vi "Get Users.vi"(3 "error in (no error)":errorcluster, 5 "Database.lvlib:Data Store.lvclass":refnum<class "Data Store.lvclass">) -> (0 "error out":errorcluster, 1 "Array":T1[](array[typedef]), 2 "Database.lvlib:Data Store.lvclass 2":refnum<class "Data Store.lvclass">)   [LabVIEW 2011, in "Database.lvlib" / "Data Store.lvclass"]
uses:
  Data Store.lvclass
  User.ctl
  Data Store.lvclass/Data Store.ctl
  <vilib>/addons/database/_DB Variant To Data/Database Variant To Data.xnode
  <vilib>/addons/database/NI_Database_API.lvlib
  Database.lvlib
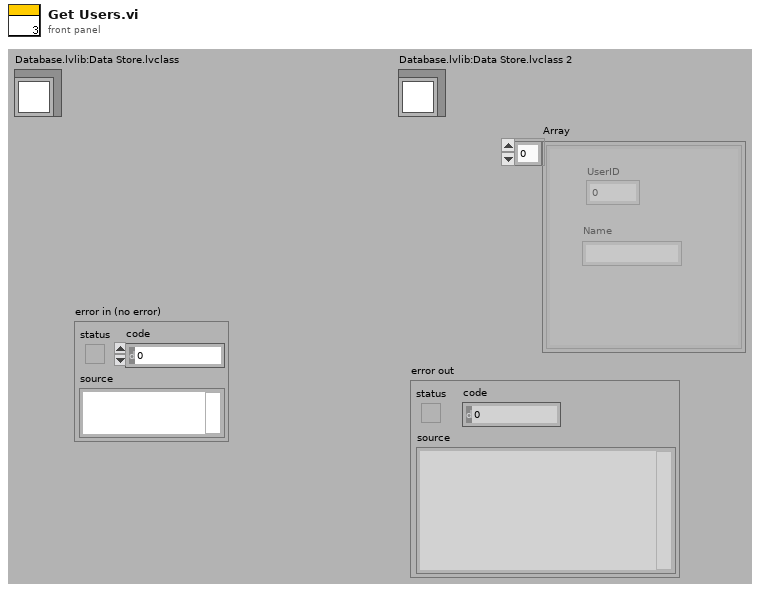
[diagram p1: front panel]
types:
  T1 = typedef "Database.lvlib/User.ctl" = cluster{"UserID":i32, "Name":string}
  T2 = typedef "NI_Database_API.lvlib/Conn ObjectReference.ctl" = refnum<k1>
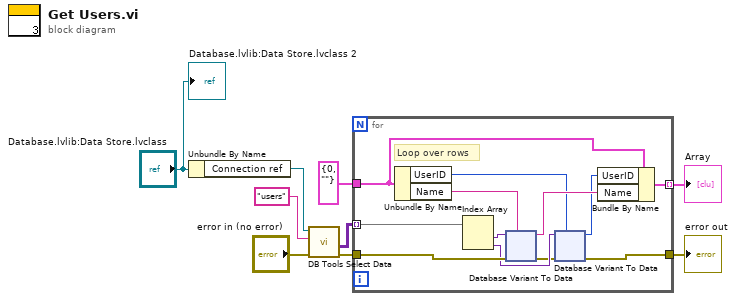
[diagram p0: block diagram]
diagram:
  n1 = Unbundle By Name("Database.lvlib:Data Store.lvclass") -> ("Connection ref"=w9:T2)
  n2 = call <vilib>:"DB Tools Select Data.vi"("error in (no error)"="error in (no error)", "table"="users", "connection reference"=w9) -> ("error out"=w6:errorcluster, "data"=w5:variant[][])  [unwired: 3 in, 1 out]
  n3 = for {
    tunnel: w6 -> [w19]
    tunnel: w5 -> [w21] mode=indexing
    tunnel: T1 {"UserID"=0, "Name"=""} ("Cluster") -> [w16]
    tunnel: [w14] -> w3 mode=indexing
    tunnel: [w15] -> w2
    # "Loop over rows"
    n4 = Unbundle By Name(w16) -> ("UserID"=w11:i32, "Name"=w13:string)
    n5 = Index Array(array=w21) -> (element #1=w20:variant, element #2=w18:variant)  [unwired: 2 in]
    n6 = xnode "Database Variant To Data"("database variant"=w20, "error in"=w19, "type"=w13) -> ("data"=w12:string, "error out"=w17:errorcluster)
    n7 = xnode "Database Variant To Data"("database variant"=w18, "error in"=w17, "type"=w11) -> ("data"=w10:i32, "error out"=w15:errorcluster)
    n8 = Bundle By Name(cluster=w16, "UserID"=w10, "Name"=w12) -> (w14:T1)
  }
  "error out" <- w2
  "Array" <- w3
  "Database.lvlib:Data Store.lvclass 2" <- "Database.lvlib:Data Store.lvclass"
